vi "05.3 Analyze and Visualize Data.vi"() -> ()   [LabVIEW 2019]
uses:
  <vilib>/DAQmx/read.llb/DAQmx Read (Analog DBL 1Chan 1Samp).vi
  <vilib>/DAQmx/miscellaneous.llb/DAQmx Fill In Error Info.vi
panel:
  out "Threshold exceeded?":bool
  out "message":string
  in  "max temperature threshold (deg C)":i8(slide) scale=15.0..50.0
  out "error out":errorcluster
  out "Current Temperature (deg C)":dbl format="%0.2f"
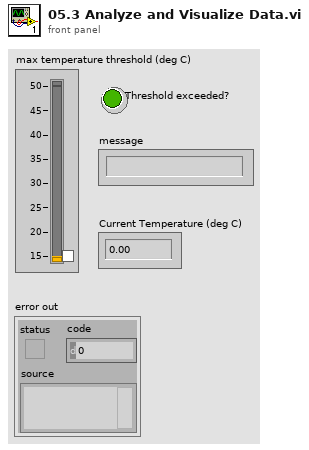
[diagram p1: front panel]
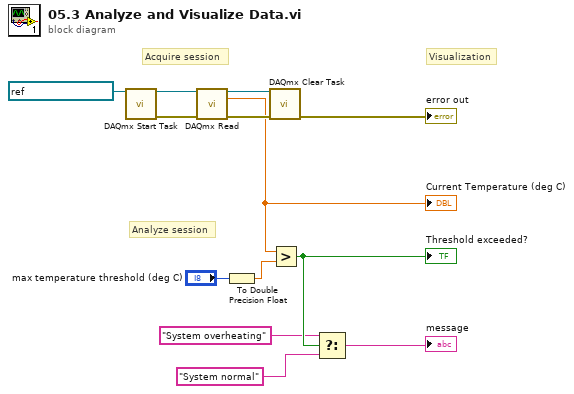
[diagram p0: block diagram]
diagram:
  # "Visualization"
  # "Analyze session"
  # "Acquire session"
  n1 = call <vilib>:"DAQmx Start Task.vi"("task/channels in"=refnum<k21> "Thermocouple") -> ("task out"=w12:refnum<k21>, "error out"=w10:errorcluster)  [unwired: 13 in]
  n2 = call-poly <vilib>:"DAQmx Read.vi"("task/channels in"=w12, "error in"=w10) -> ("task out"=w11:refnum<k21>, "data"=w7:dbl, "error out"=w9:errorcluster)  [unwired: 11 in]
  "Current Temperature (deg C)" <- w7
  n3 = To Double Precision Float(number="max temperature threshold (deg C)") -> (double precision float=w1:dbl)
  n4 = call <vilib>:"DAQmx Clear Task.vi"("task in"=w11, "error in"=w9) -> ("error out"=→"error out":errorcluster)  [unwired: 13 in]
  n5 = Greater?(x=w7, y=w1) -> (0:w6:bool)
  "Threshold exceeded?" <- w6
  n6 = Select(t="System overheating", s=w6, f="System normal") -> (s? t:f=→"message":string)
